vi "test Scheduled Loopback.vi"(8 "error in":errorcluster, 11 "TestCase in":refnum<class "Single Board Loopback.lvclass">) -> (0 "error out":errorcluster, 3 "TestCase out":refnum<class "Single Board Loopback.lvclass">)   [LabVIEW 2020, in "Single Board Loopback.lvclass"]
uses:
  Single Board Loopback.lvclass
  C:/dev/git/niveristand-custom-device-testing-tools/VeriStandTestCase/VeriStandTestCase.lvclass
  <vilib>/numeric/Random Number (Range) U64.vi
  <vilib>/numeric/sub_Random U32.vi
  <vilib>/addons/_JKI Toolkits/VI Tester/TestCase.llb/TestCase.lvclass
  niveristand-custom-device-testing-tools/VeriStandTestUtilities/VeriStandTestUtilities.lvlib
  C:/Program Files (x86)/National Instruments/LabVIEW 2020/vi.lib/addons/_JKI Toolkits/VI Tester/TestCase.llb/TestCase.lvclass
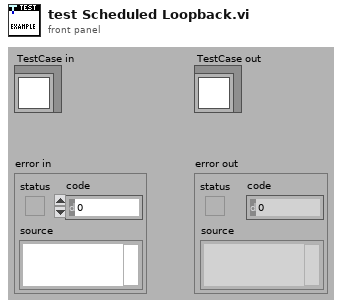
[diagram p1: front panel]
types:
  T1 = typedef "NI_VS Workspace ExecutionAPI.lvlib/WorkspaceAPI.ctl" = refnum<k24>
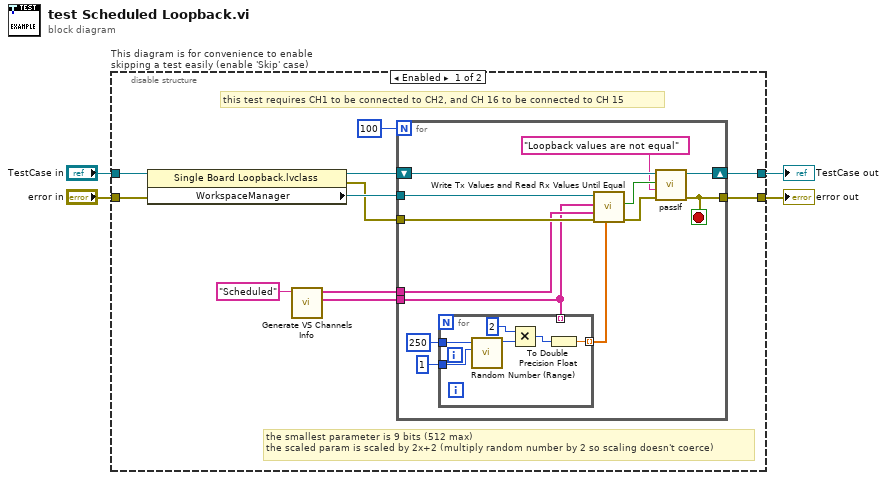
[diagram p0: block diagram]
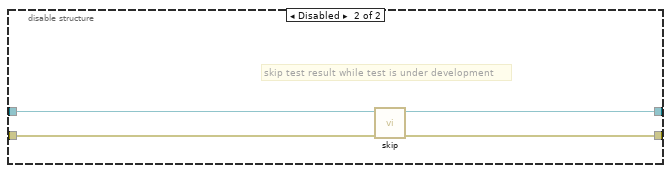
[diagram p2: hidden frame]
diagram:
  n1 = disable-structure "This diagram is for convenience to enable skipping a test easily (enable 'Skip' case)" shown="Enabled" {
    disable-tunnel: "TestCase in" -> [w10 w38]
    disable-tunnel: [w8 w36] -> w1
    disable-tunnel: [w7 w37] -> w3
    disable-tunnel: "error in" -> [w9 w35]
    frame Enabled {
      # "this test requires CH1 to be connected to CH2, and CH 16 to be connected to CH 15"
      # "the smallest parameter is 9 bits (512 max)\nthe scaled param is scaled by 2x+2 (multiply random number by 2 so scaling doesn't coerce)"
      n2 = property class="Single Board Loopback.lvclass"(reference=w10, error in=w9) -> (reference out=w12:refnum<class "Single Board Loopback.lvclass">, error out=w13:errorcluster, "WorkspaceManager"=w14:T1)
      n3 = call "Generate VS Channels Info.vi"("Transfer Type"="Scheduled") -> ("Tx Channels Array"=w6:string[], "Rx Channels Array"=w15:string[])  [unwired: 6 in, 3 out]
      n4 = for {
        N: 100 -> [_]
        tunnel: w15 -> [w17]
        tunnel: w14 -> [w28]
        tunnel: w13 -> [w27]
        tunnel: w6 -> [w16]
        shift-right: [w24] -> w8
        shift-left: w12 -> [w25]
        tunnel: [w23] -> w7
        stop <- w23 stop-if-true
        n5 = for {
          tunnel: [w33] -> w18 mode=indexing
          tunnel: u64 250 ("upper bound (100)") -> [w32]
          tunnel: u64 1 ("upper bound (100)") -> [w31]
          tunnel: w16 -> [_] mode=indexing
          n6 = call-poly <vilib>:"Random Number (Range).vi"("lower bound (0)"=w31, "upper bound (100)"=w32) -> ("number"=w34:u64)  [unwired: 9 in]
          n7 = Multiply(x=u64 2, y=w34) -> (x*y=w30:u64)
          n8 = To Double Precision Float(number=w30) -> (double precision float=w33:dbl)
        }
        n9 = call "Write Tx Values and Read Rx Values Until Equal.vi"("Tx values"=w18, "error in"=w27, "Rx aliases"=w17, "Tx aliases"=w16, "workspace manager in"=w28) -> ("error out"=w26:errorcluster, "values equal"=w22:bool)  [unwired: 4 in, 1 out]
        n10 = call-dynamic "passIf.vi"("error in (no error)"=w26, "message (\"\")"="Loopback values are not equal" ("message (\"\")"), "pass"=w22, "TestCase in"=w25) -> ("error out"=w23:errorcluster, "TestCase out"=w24:refnum<class "Single Board Loopback.lvclass">)  [unwired: 6 in]
      }
    }
    frame Disabled {
      # "skip test result while test is under development"
      n11 = call <vilib>:"skip.vi"("error in (no error)"=w35, "TestCase in"=w38) -> ("error out"=w37:errorcluster, "TestCase out"=w36:refnum<class "Single Board Loopback.lvclass">)  [unwired: 8 in]
    }
  }
  "error out" <- w3
  "TestCase out" <- w1
